vi "draw.vi"(8 "error in (no error)":errorcluster, 11 "Kreisquadrant in":refnum<class "Kreisquadrant.lvclass">) -> (0 "error out":errorcluster, 2 "element":cluster{"x":dbl[], "y":dbl[]}, 3 "Kreisquadrant out":refnum<class "Kreisquadrant.lvclass">)   [LabVIEW 2019, in "Kreisquadrant.lvclass"]
uses:
  Kreisquadrant.lvclass
  mode_Q.ctl
  Kreisquadrant.lvclass/Kreisquadrant.ctl
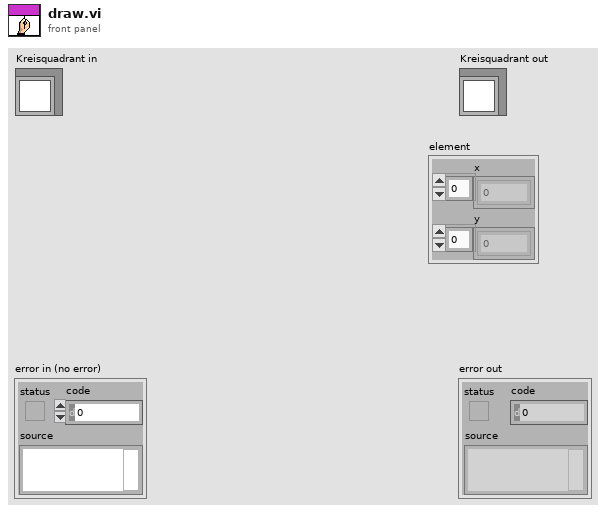
[diagram p1: front panel]
types:
  T1 = typedef "mode_Q.ctl" = enum16{"init", "get"}
  T2 = typedef "Quadrant.ctl" = enum16{"oben_rechts", "oben_links", "unten_links", "unten_rechts"}
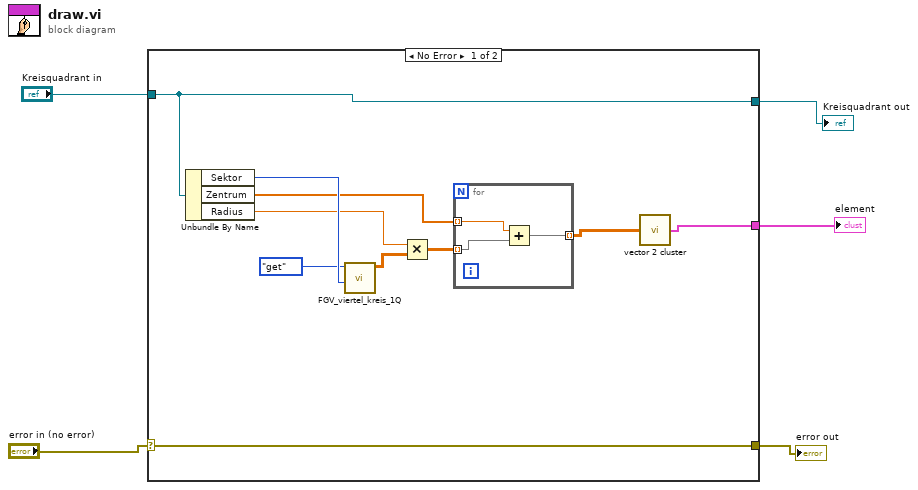
[diagram p0: block diagram]
diagram:
  n1 = case shown="No Error" "error in (no error)" {
    selector: "error in (no error)" -> [w15 w19]
    tunnel: [w15 w19] -> w4
    tunnel: [w14 w20] -> w3
    tunnel: "Kreisquadrant in" -> [w14 w20]
    tunnel: [w6 _] -> w1
    frame No Error {
      n2 = Unbundle By Name(w14) -> ("Sektor"=w13:T2, "Zentrum"=w8:dbl[], "Radius"=w10:dbl)
      n3 = call "FGV_viertel_kreis_1Q.vi"("Sektor"=w13, "mode"=mode_Q."get") -> ("Q"=w11:dbl[][])  [unwired: 7 in, 2 out]
      n4 = Multiply(x=w10, y=w11) -> (x*y=w9:dbl[][])
      n5 = for {
        tunnel: w9 -> [w18] mode=indexing
        tunnel: w8 -> [w17] mode=indexing
        tunnel: [w16] -> w7 mode=indexing
        n6 = Add(x=w17, y=w18) -> (x+y=w16:dbl[])
      }
      n7 = call "vector 2 cluster.vi"("coordinates"=w7) -> (0:w6:cluster{"x":dbl[], "y":dbl[]})
    }
    frame Error {
    }
  }
  "error out" <- w4
  "Kreisquadrant out" <- w3
  "element" <- w1
